vi "main.vi"() -> ()   [LabVIEW 2021]
panel:
  in  "Attenuation":string(combo)
  in  "Level":dbl
  in  "Cmos":string(combo)
  in  "Duty":dbl
  in  "Modulation":string(combo)
  in  "Frequency":dbl
  in  "Range":string(combo)
  in  "Offset":dbl
  in  "Counter":string(combo)
  out "error in":errorcluster
  out "error out":errorcluster
  in  "Function type":string(combo)
  in  "close":bool=TRUE
  out "VISA resource name out":refnum<visa-resource-name>
  in  "open":bool=TRUE
  in  "VISA resource name":refnum<visa-resource-name>
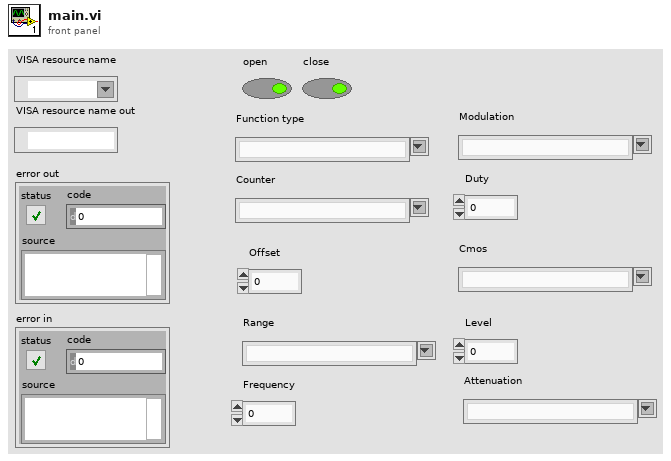
[diagram p1: front panel]
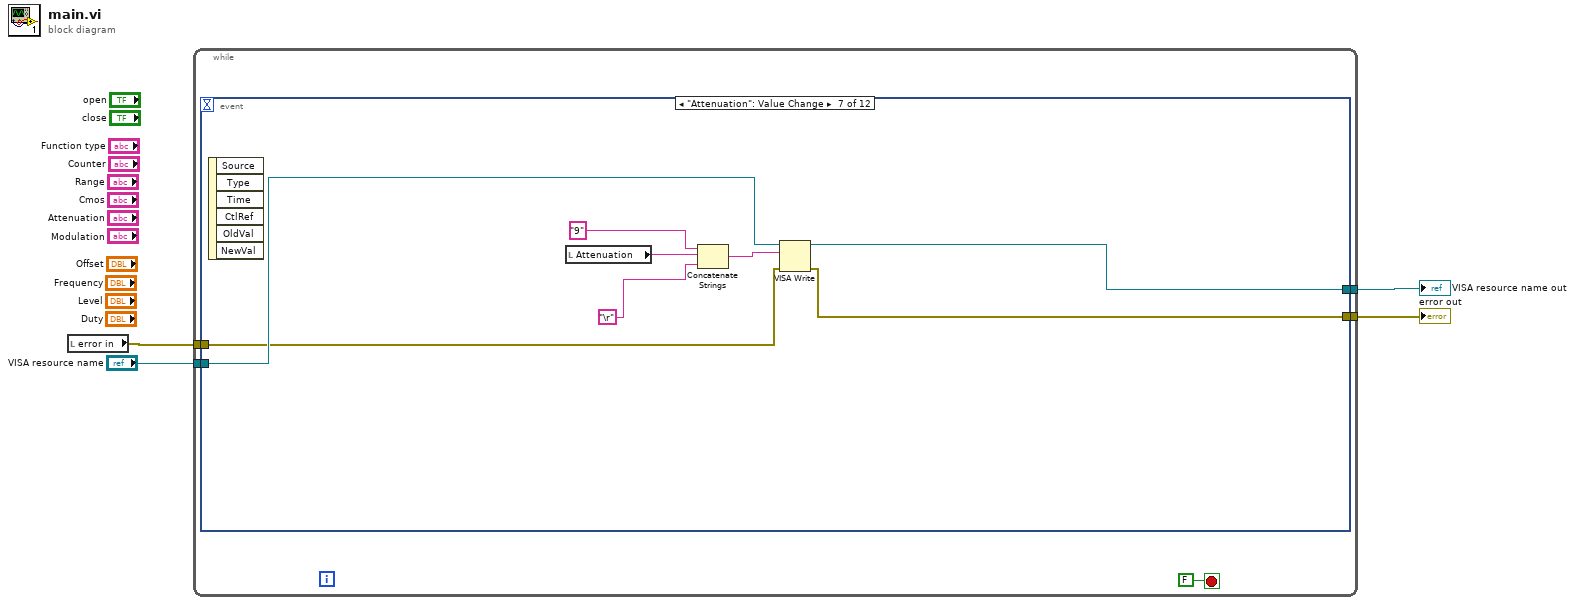
[diagram p0: block diagram]
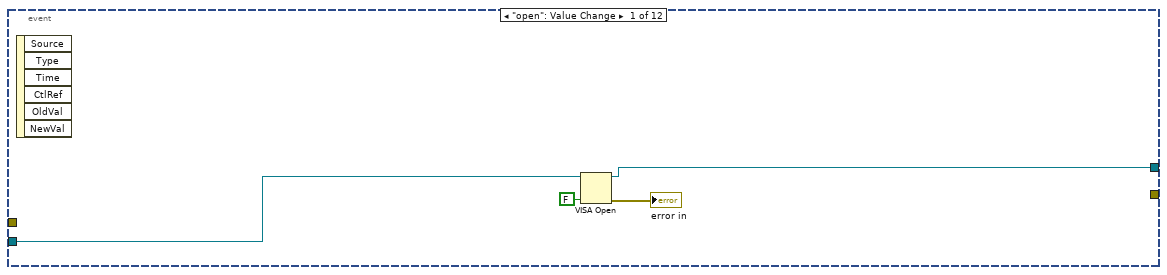
[diagram p2: hidden frame]
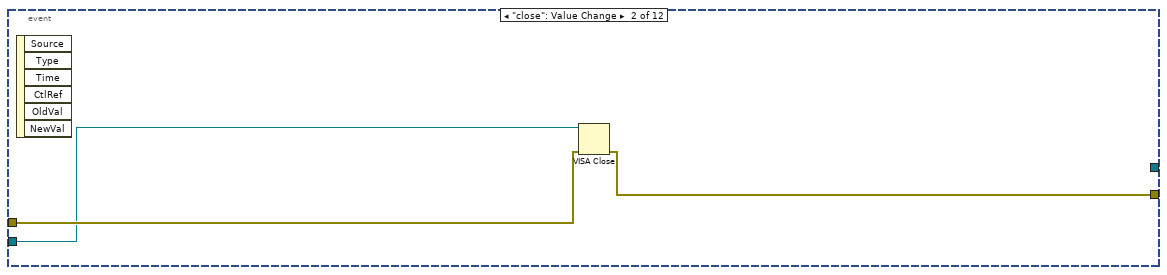
[diagram p3: hidden frame]
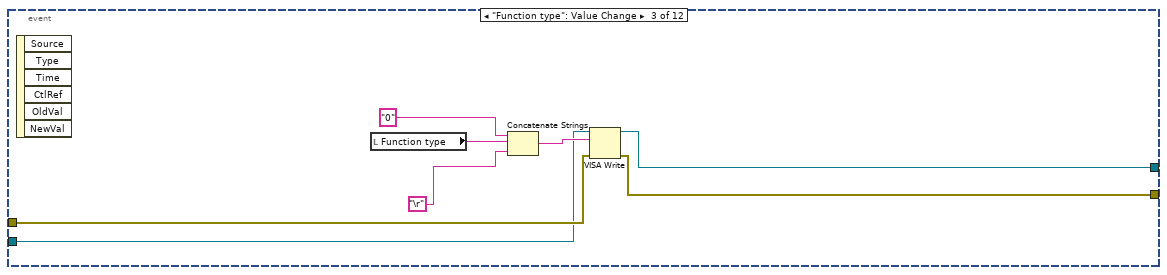
[diagram p4: hidden frame]
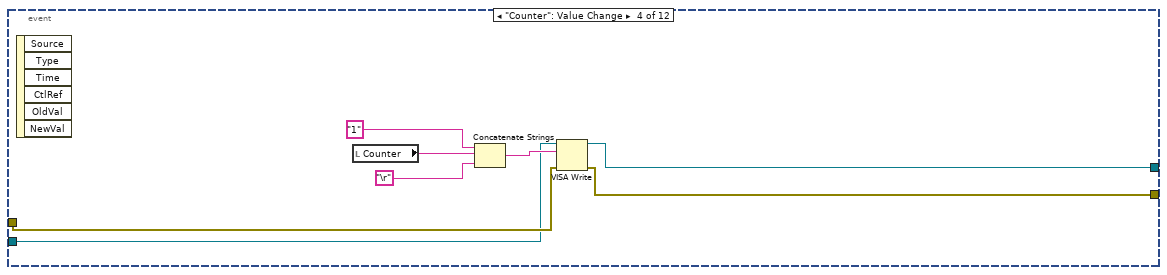
[diagram p5: hidden frame]
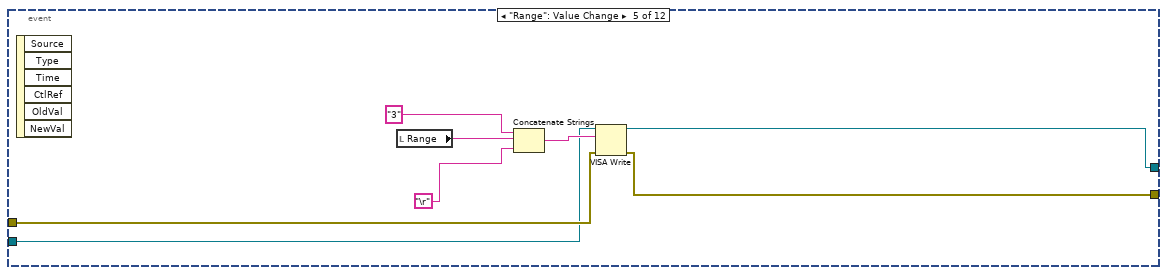
[diagram p6: hidden frame]
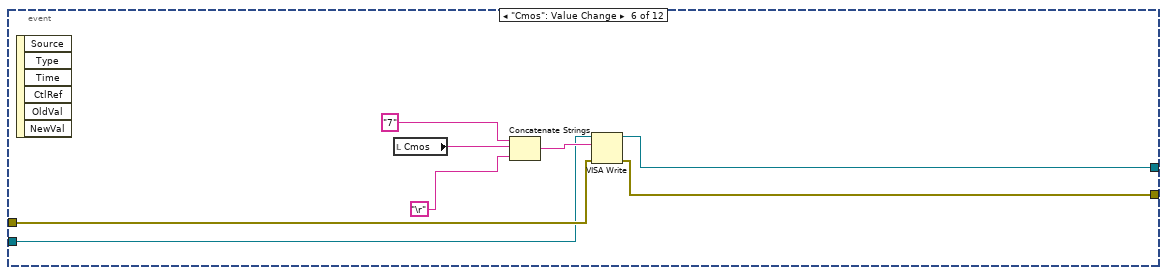
[diagram p7: hidden frame]
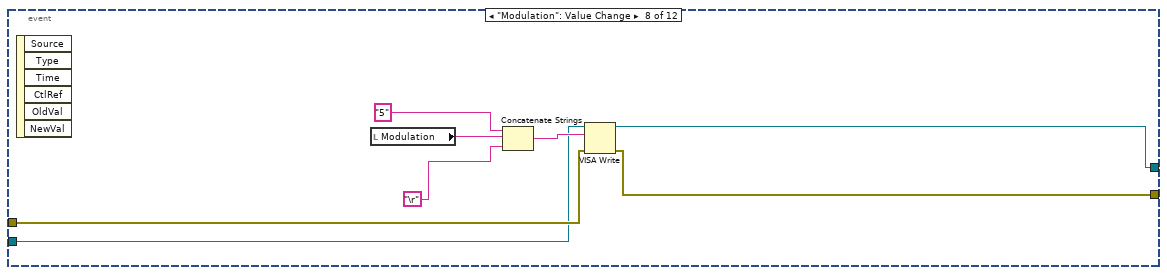
[diagram p8: hidden frame]
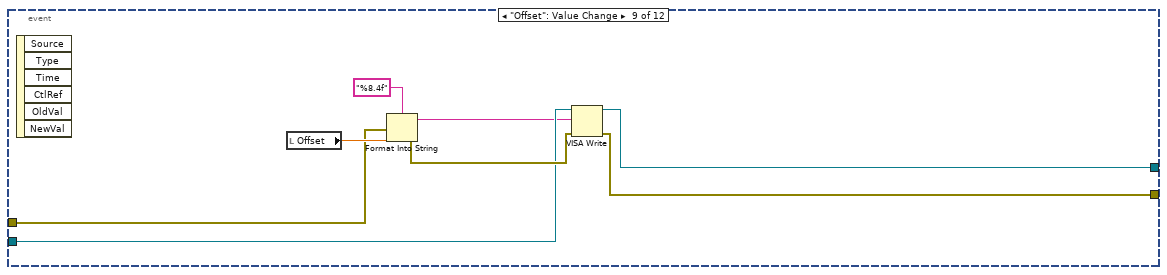
[diagram p9: hidden frame]
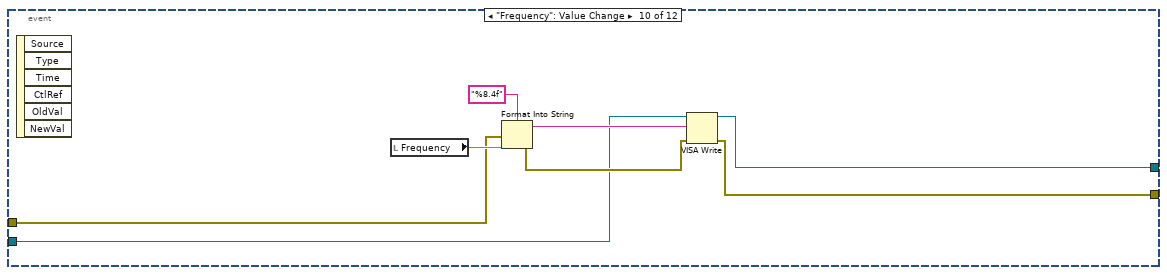
[diagram p10: hidden frame]
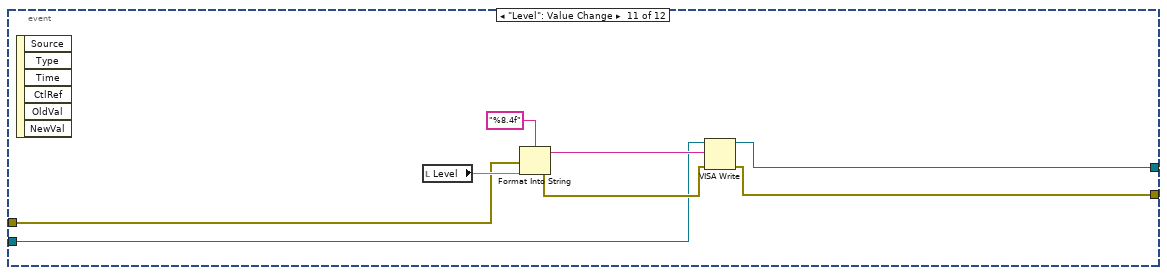
[diagram p11: hidden frame]
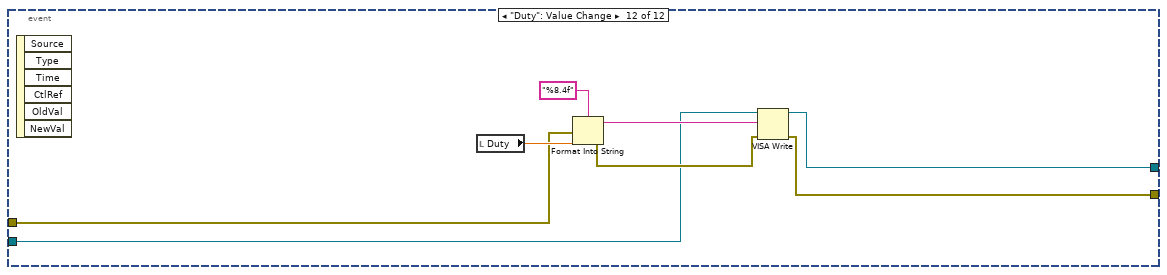
[diagram p12: hidden frame]
diagram:
  n1 = local read "error in"() -> (w4:errorcluster)
  n2 = while {
    tunnel: w4 -> [w8]
    tunnel: [w7] -> w3
    tunnel: "VISA resource name" -> [w6]
    tunnel: [w5] -> w1
    stop <- FALSE ("stop") stop-if-true
    n3 = event shown="[6] \"Attenuation\": Value Change" {
      selector: _ -> [_ _ _ _ _ _ _ _ _ _ _ _]
      dyn-events: _ -> [_ _ _ _ _ _ _ _ _ _ _ _]
      timeout: _ -> [_ _ _ _ _ _ _ _ _ _ _ _]
      tunnel: w8 -> [_ w16 w20 w28 w36 w44 w51 w60 w70 w76 w84 w92]
      tunnel: [_ w15 w19 w27 w33 w42 w49 w57 w68 w73 w82 w89] -> w7
      tunnel: w6 -> [w11 w14 w18 w25 w35 w43 w52 w59 w67 w75 w83 w91]
      tunnel: [w10 _ w17 w26 w34 w41 w50 w58 w65 w74 w81 w90] -> w5
      event "open": Value Change {
        n4 = event-data() -> ()  [unwired: 1 in, 6 out]
        n5 = VISA Open(duplicate session (F)=FALSE, VISA resource name=w11) -> (VISA resource name=w10:refnum<visa-resource-name>, error out=→"error in":errorcluster)  [unwired: 3 in]
      }
      event "close": Value Change {
        n6 = event-data() -> ()  [unwired: 1 in, 6 out]
        n7 = VISA Close(VISA resource name=w14, error in (no error)=w16) -> (error out=w15:errorcluster)
      }
      event "Function type": Value Change {
        n8 = event-data() -> ()  [unwired: 1 in, 6 out]
        n9 = local read "Function type"() -> (w24:string)
        n10 = Concatenate Strings("0" ("string"), w24, "\r") -> (w22:string)
        n11 = VISA Write(VISA resource name=w18, write buffer=w22, error in (no error)=w20) -> (VISA resource name out=w17:refnum<visa-resource-name>, error out=w19:errorcluster)  [unwired: 1 out]
      }
      event "Counter": Value Change {
        n12 = event-data() -> ()  [unwired: 1 in, 6 out]
        n13 = local read "Counter"() -> (w29:string)
        n14 = Concatenate Strings("1" ("string"), w29, "\r") -> (w31:string)
        n15 = VISA Write(VISA resource name=w25, write buffer=w31, error in (no error)=w28) -> (VISA resource name out=w26:refnum<visa-resource-name>, error out=w27:errorcluster)  [unwired: 1 out]
      }
      event "Range": Value Change {
        n16 = event-data() -> ()  [unwired: 1 in, 6 out]
        n17 = local read "Range"() -> (w37:string)
        n18 = Concatenate Strings("3" ("string"), w37, "\r") -> (w39:string)
        n19 = VISA Write(VISA resource name=w35, write buffer=w39, error in (no error)=w36) -> (VISA resource name out=w34:refnum<visa-resource-name>, error out=w33:errorcluster)  [unwired: 1 out]
      }
      event "Cmos": Value Change {
        n20 = event-data() -> ()  [unwired: 1 in, 6 out]
        n21 = local read "Cmos"() -> (w45:string)
        n22 = Concatenate Strings("7" ("string"), w45, "\r") -> (w47:string)
        n23 = VISA Write(VISA resource name=w43, write buffer=w47, error in (no error)=w44) -> (VISA resource name out=w41:refnum<visa-resource-name>, error out=w42:errorcluster)  [unwired: 1 out]
      }
      event "Attenuation": Value Change {
        n24 = event-data() -> ()  [unwired: 1 in, 6 out]
        n25 = local read "Attenuation"() -> (w53:string)
        n26 = Concatenate Strings("9" ("string"), w53, "\r") -> (w55:string)
        n27 = VISA Write(VISA resource name=w52, write buffer=w55, error in (no error)=w51) -> (VISA resource name out=w50:refnum<visa-resource-name>, error out=w49:errorcluster)  [unwired: 1 out]
      }
      event "Modulation": Value Change {
        n28 = event-data() -> ()  [unwired: 1 in, 6 out]
        n29 = local read "Modulation"() -> (w61:string)
        n30 = Concatenate Strings("5" ("string"), w61, "\r") -> (w63:string)
        n31 = VISA Write(VISA resource name=w59, write buffer=w63, error in (no error)=w60) -> (VISA resource name out=w58:refnum<visa-resource-name>, error out=w57:errorcluster)  [unwired: 1 out]
      }
      event "Offset": Value Change {
        n32 = event-data() -> ()  [unwired: 1 in, 6 out]
        n33 = local read "Offset"() -> (w72:dbl)
        n34 = Format Into String(format string="%8.4f", error in=w70, w72) -> (resulting string=w66:string, error out=w69:errorcluster)  [unwired: 1 in]
        n35 = VISA Write(VISA resource name=w67, write buffer=w66, error in (no error)=w69) -> (VISA resource name out=w65:refnum<visa-resource-name>, error out=w68:errorcluster)  [unwired: 1 out]
      }
      event "Frequency": Value Change {
        n36 = event-data() -> ()  [unwired: 1 in, 6 out]
        n37 = local read "Frequency"() -> (w80:dbl)
        n38 = Format Into String(format string="%8.4f", error in=w76, w80) -> (resulting string=w77:string, error out=w78:errorcluster)  [unwired: 1 in]
        n39 = VISA Write(VISA resource name=w75, write buffer=w77, error in (no error)=w78) -> (VISA resource name out=w74:refnum<visa-resource-name>, error out=w73:errorcluster)  [unwired: 1 out]
      }
      event "Level": Value Change {
        n40 = event-data() -> ()  [unwired: 1 in, 6 out]
        n41 = local read "Level"() -> (w88:dbl)
        n42 = Format Into String(format string="%8.4f", error in=w84, w88) -> (resulting string=w85:string, error out=w86:errorcluster)  [unwired: 1 in]
        n43 = VISA Write(VISA resource name=w83, write buffer=w85, error in (no error)=w86) -> (VISA resource name out=w81:refnum<visa-resource-name>, error out=w82:errorcluster)  [unwired: 1 out]
      }
      event "Duty": Value Change {
        n44 = event-data() -> ()  [unwired: 1 in, 6 out]
        n45 = local read "Duty"() -> (w96:dbl)
        n46 = Format Into String(format string="%8.4f", error in=w92, w96) -> (resulting string=w93:string, error out=w94:errorcluster)  [unwired: 1 in]
        n47 = VISA Write(VISA resource name=w91, write buffer=w93, error in (no error)=w94) -> (VISA resource name out=w90:refnum<visa-resource-name>, error out=w89:errorcluster)  [unwired: 1 out]
      }
    }
  }
  "error out" <- w3
  "VISA resource name out" <- w1
